vi "ClassPanel.vi"(8 "error in (no error)":errorcluster caption="entrée d'erreur (pas d'erreur)", 11 "AndorSpectro.lvclass":refnum<class "AndorSpectro.lvclass">) -> (0 "error out":errorcluster caption="sortie d'erreur", 3 "AndorSpectro.lvclass Out":refnum<class "AndorSpectro.lvclass">)   [LabVIEW 2019, in "AndorSpectro.lvclass"]
uses:
  AndorSpectro.lvclass
  C:/Programmes Labview/LabscanV1A/DevicesClass/BaseDevice/BaseDevice.lvclass
  <userlib>/ATSpectrograph/GUI/AndorNoiseCorr.ctl
  <userlib>/atmcd32d.llb/AndorCapabilities typedef.ctl
  <userlib>/atmcd32d.llb/Shutter_type typedef.ctl
  <userlib>/atmcd32d.llb/Shutter_mode typedef.ctl
  <userlib>/atmcd32d.llb/AcquisitionMode_mode typedef.ctl
  <userlib>/atmcd32d.llb/ReadMode_mode typedef.ctl
  <userlib>/atmcd32d.llb/Error Code Enum typedef.ctl
  BaseDevice/BaseDevice.lvclass/BaseDevice.ctl
  <userlib>/atmcd32d.llb/TriggerMode_mode typedef.ctl
  BaseDevice/ClassQueueMess.ctl
  <userlib>/atmcd32d.llb/HSSpeed_type typedef.ctl
  AndorSpectro.lvclass/AndorSpectro.ctl
  BaseDevice/Accessor/GetBaseDataPath.vi
  BaseDevice/Accessor/GetClassEvent.vi
  <userlib>/ATSpectrograph/atspectrograph.lvlib
panel:
  out "exposure":sgl format="%.4f"
  out "Top Wl":sgl=100.0 caption="Top Wl. (nm)" min=0 max=3000 step=0.01
  out "Bot Wl":sgl=100.0 caption="Bot Wl. (nm)" min=0 max=3000 step=0.01
  out "BaseDataPath":path
  out "Background":i32[][](array[numeric])
  out "AndorMainQ":refnum<queue>
  out "Wavelength":sgl
  out "CalValues":sgl[](array[numeric])
  out "Detector offset":i32
  out "grating out":i32
  out "Grating offset":i32
  out "gain":sgl format="%.2f"
  out "information":i32
  out "caps":T1
  in  "X Start":i32=1 min=1 max=1023 step=1
  in  "X End":i32=1024 min=2 max=1024 step=1
  in  "AndorTabs":enum32{"Main Controls", "Settings", "Data"}(tab)
  in  "Shutter":bool
  in  "DIsOnCLose":bool=TRUE caption="Dis.On Close"
  in  "AccDone":u16 caption="Acq. Done"
  in  "Stop Acq":bool
  in  "Con/Disc.":bool
  in  "Gain":i32(ring) caption="Device Name" items=["1.0(x)", "1.7(x)"]
  in  "Image Mode":bool
  in  "AquireImage":bool caption="MiseAJour"
  out "AcqTime":sgl caption="Acq. Time (s)" format="%#.4f"
  in  "IntegTime":u32=100 caption="Integration\nTime (ms)" min=1 max=100000 step=1
  in  "Accumulation":u16=1 min=1 max=256 step=1
  out "Temp °C":i32
  in  "Cooler":bool
  in  "Save Data":bool caption="Save\nData"
  in  "Cont. Acq.":bool caption="Cont.Acq."
  out "Stable":bool
  in  "Setp. °C":i32=-80
  out "Aquiring":bool
  in  "Save Bckgnd":bool caption="Save as \nBckgnd"
  in  "Backgnd Mode":T2
  in  "SetAreas":bool caption="MiseAJour"
  in  "Y Bins":i32=1 min=1 max=256 step=1
  out "areas":i32[][](array[numeric])=[[1], [1], [1], [1024], [256], [1], [256]]
  in  "HS":u16(ring) caption="Hor. Spd." items=["100kHz@16bit", "50kHz@16bit", "33kHz@16bit"]
  in  "VS":u16(ring)=1 caption="Vert. Spd (us)" items=["[8.25]", "16.25", "32.25", "64.25"]
  in  "Y End":i32=256 min=2 max=256 step=1
  in  "Y Start":i32=1 min=1 max=255 step=1
  in  "ShutterMode":u16(ring) items=["IDUS_Shutter", "Ext Shutter"]
  out "Start(nm)":sgl=1.0 min=1 max=255 step=1
  out "End(nm)":sgl=1.0 min=1 max=255 step=1
  out "WaveBands":T3(array[cluster]) {"WB End" min=1 max=255 step=1; "WB Start" min=1 max=255 step=1}
  in  "DelWB":bool caption="MiseAJour"
  in  "AddWB":bool caption="MiseAJour"
  in  "WB End":i32=256 min=2 max=1024 step=1
  in  "WB Start":i32=1 min=1 max=1023 step=1
  in  "NoiseWindow":bool caption="Noise Window"
  in  "Cosmic Filter":bool
  in  "MainProgQ":refnum<queue>
  in  "MainProgQEvent":refnum<user-event>
  in  "Acq":bool
  in  "Stop":bool
  out "Init Program":bool
  # "Andor Camera"
  # "this MUST labeled with class name"
  # "this MUST be present and labeled \"Stop\" and \"Acq\""
  # "Single Acq"
  # "Area#"
  # "X Origin"
  # "Y Origin"
  # "X Size"
  # "Y Size"
  # "X Bin"
  # "Y Bin"
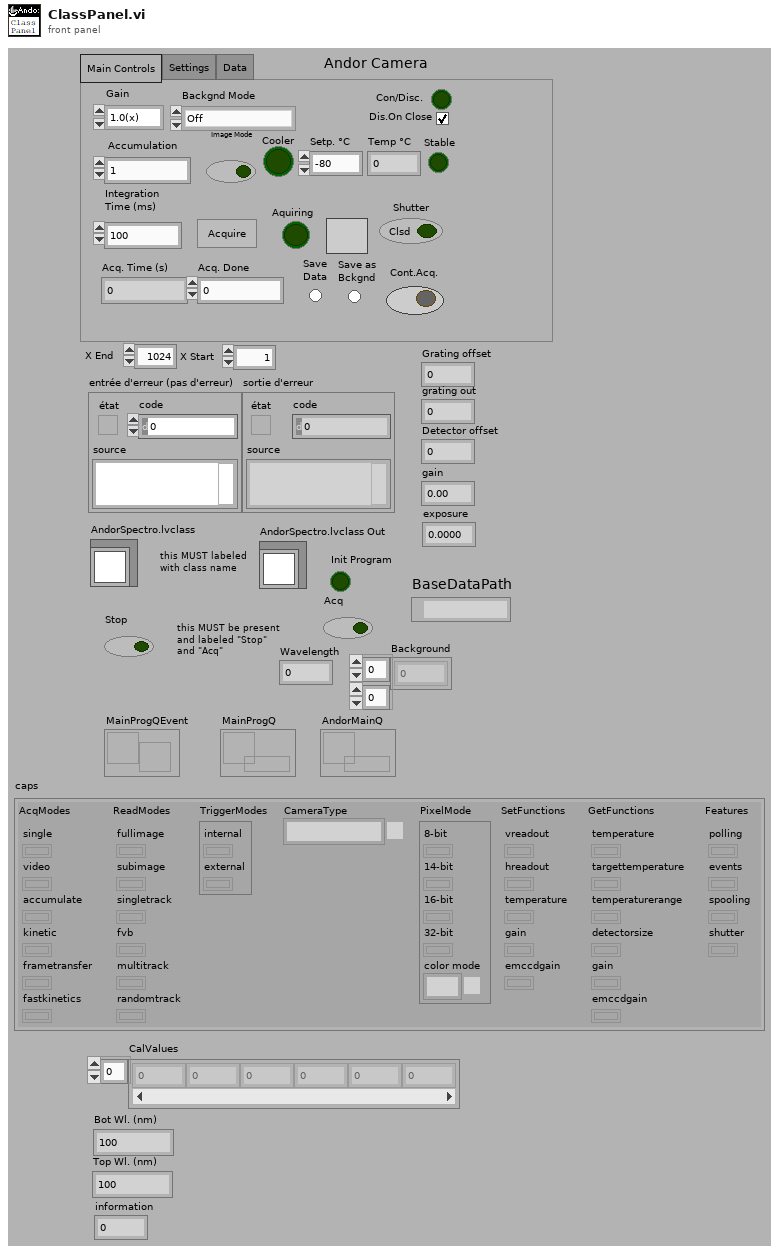
[diagram p1: front panel]
types:
  T1 = typedef "AndorCapabilities typedef.ctl" = cluster{"AcqModes":cluster{"single":bool, "video":bool, "accumulate":bool, "kinetic":bool, "frametransfer":bool, "fastkinetics":bool}, "ReadModes":cluster{"fullimage":bool, "subimage":bool, "singletrack":bool, "fvb":bool, "multitrack":bool, "randomtrack":bool}, "TriggerModes":cluster{"internal":bool, "external":bool}, "CameraType":enum32{"PDA", "iXon", "ICCD", "EMCCD", "CCD", "iStar", "third party camera", "iDus", "Newton", "Surcam", "USB ICCD", "Luca", "Reserved", "iKon", "InGaAs", "iVac", "Unprogrammed", "Clara", "USB iStar", "SimCam", "Neo", "iXon Ultra", "Volmos", "iVac Ultra"}, "PixelMode":cluster{"8-bit":bool, "14-bit":bool, "16-bit":bool, "32-bit":bool, "color mode":enum16{"Mono", "RGB", "CMY"}}, "SetFunctions":cluster{"vreadout":bool, "hreadout":bool, "temperature":bool, "gain":bool, "emccdgain":bool}, "GetFunctions":cluster{"temperature":bool, "targettemperature":bool, "temperaturerange":bool, "detectorsize":bool, "gain":bool, "emccdgain":bool}, "Features":cluster{"polling":bool, "events":bool, "spooling":bool, "shutter":bool}}
  T2 = typedef "AndorNoiseCorr.ctl" = enum16{"Off", "Selected Curve", "One For Every Acq"}
  T3 = cluster{"WB Start":i32, "WB End":i32, "Active":bool}[]
  T4 = cluster{"Message":string, "Data":variant, "Code":i32}
  T5 = typedef "Shutter_mode typedef.ctl" = enum16{"Auto", "Open", "Close", "N/A (3)", "Open FVB Series", "Open Any Series"}
  T6 = typedef "Shutter_type typedef.ctl" = enum16{"TTL Low", "TTL High"}
  T7 = typedef "AcquisitionMode_mode typedef.ctl" = enum16{"Reserved (0)", "Single Scan", "Accumulate", "Kinetics", "Fast Kinetics", "Run Till Abort", "Reserved (6)", "Reserved (7)", "Reserved (8)", "Time Delayed Integration"}
  T8 = typedef "ReadMode_mode typedef.ctl" = enum16{"Full Vertical Binning", "Multi-Track", "Random-Track", "Single-Track", "Image"}
  T9 = typedef "Error Code Enum typedef.ctl" = enum32{"N/A (0)", "DRV_ERROR_CODES", "DRV_SUCCESS", "DRV_VXDNOTINSTALLED", "DRV_ERROR_SCAN", "DRV_ERROR_CHECK_SUM", "DRV_ERROR_FILELOAD", "DRV_UNKNOWN_FUNC", "DRV_ERROR_VXD_INIT", "DRV_ERROR_ADDRESS", "DRV_ERROR_PAGELOCK", "DRV_ERROR_PAGEUNLOCK", "DRV_ERROR_BOARDTEST", "DRV_ERROR_ACK", "DRV_ERROR_UP_FIFO", "DRV_ERROR_PATTERN", "N/A (16)", "DRV_ACQUISITION_ERRORS", "DRV_ACQ_BUFFER", "DRV_ACQ_DOWNFIFO_FULL", "DRV_PROC_UNKONWN_INSTRUCTION", "DRV_ILLEGAL_OP_CODE", "DRV_KINETIC_TIME_NOT_MET", "DRV_ACCUM_TIME_NOT_MET", "DRV_NO_NEW_DATA", "N/A (25)", "DRV_SPOOLERROR", "N/A (27)", "N/A (28)", "N/A (29)", "N/A (30)", "N/A (31)", "N/A (32)", "DRV_TEMPERATURE_CODES", "DRV_TEMPERATURE_OFF", "DRV_TEMPERATURE_NOT_STABILIZED", "DRV_TEMPERATURE_STABILIZED", "DRV_TEMPERATURE_NOT_REACHED", "DRV_TEMPERATURE_OUT_RANGE", "DRV_TEMPERATURE_NOT_SUPPORTED", "DRV_TEMPERATURE_DRIFT", "N/A (41)", "N/A (42)", "N/A (43)", "N/A (44)", "N/A (45)", "N/A (46)", "N/A (47)", "N/A (48)", "DRV_GENERAL_ERRORS", "DRV_INVALID_AUX", "DRV_COF_NOTLOADED", "DRV_FPGAPROG", "DRV_FLEXERROR", "DRV_GPIBERROR", "N/A (55)", "N/A (56)", "N/A (57)", "N/A (58)", "N/A (59)", "N/A (60)", "N/A (61)", "N/A (62)", "N/A (63)", "DRV_DATATYPE", "DRV_DRIVER_ERRORS", "DRV_P1INVALID", "DRV_P2INVALID", "DRV_P3INVALID", "DRV_P4INVALID", "DRV_INIERROR", "DRV_COFERROR", "DRV_ACQUIRING", "DRV_IDLE", "DRV_TEMPCYCLE", "DRV_NOT_INITIALIZED", "DRV_P5INVALID", "DRV_P6INVALID", "DRV_INVALID_MODE", "DRV_INVALID_FILTER", "DRV_I2CERRORS", "DRV_I2CDEVNOTFOUND", "DRV_I2CTIMEOUT", "DRV_P7INVALID", "N/A (84)", "N/A (85)", "N/A (86)", "N/A (87)", "N/A (88)", "N/A (89)", "DRV_IOCERROR", "DRV_VRMVERSIONERROR"}
  T10 = typedef "HSSpeed_type typedef.ctl" = enum16{"EM Amp", "Conventional Amp"}
  T11 = typedef "TriggerMode_mode typedef.ctl" = enum16{"Internal", "External", "N/A (2)", "N/A (3)", "N/A (4)", "N/A (5)", "External Start"}
  T12 = typedef "ClassQueueMess.ctl" = u16
  T13 = cluster{"wavelength out":sgl, "calibrationValuesOut":sgl[], "gain":sgl, bool}
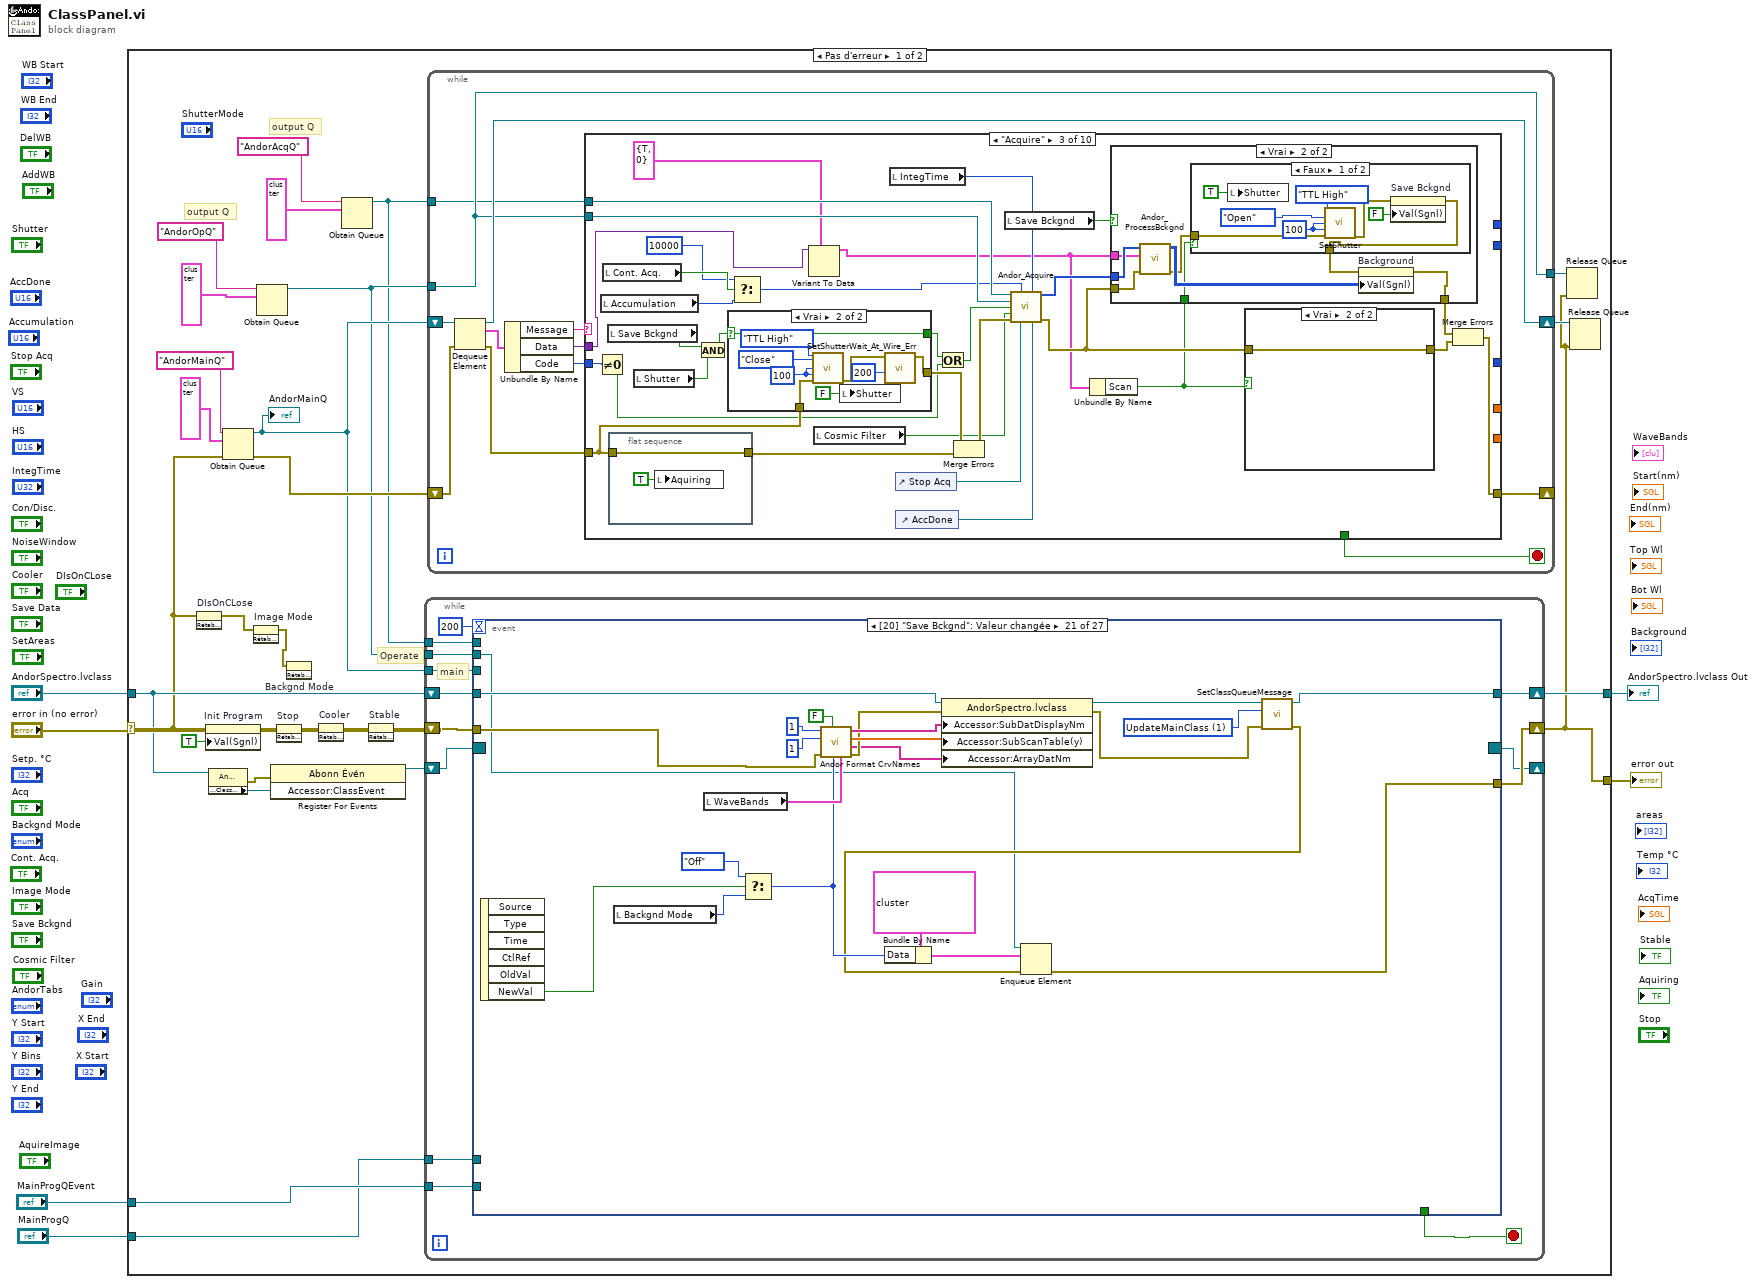
[diagram p0: block diagram]
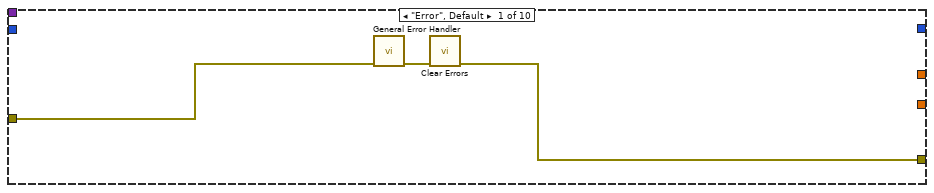
[diagram p2: hidden frame]
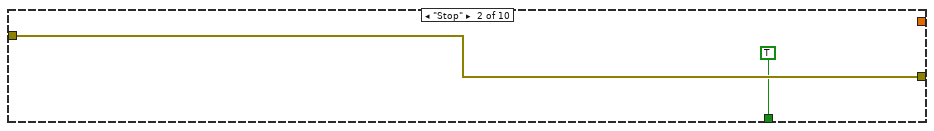
[diagram p3: hidden frame]
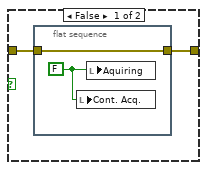
[diagram p4: hidden frame]
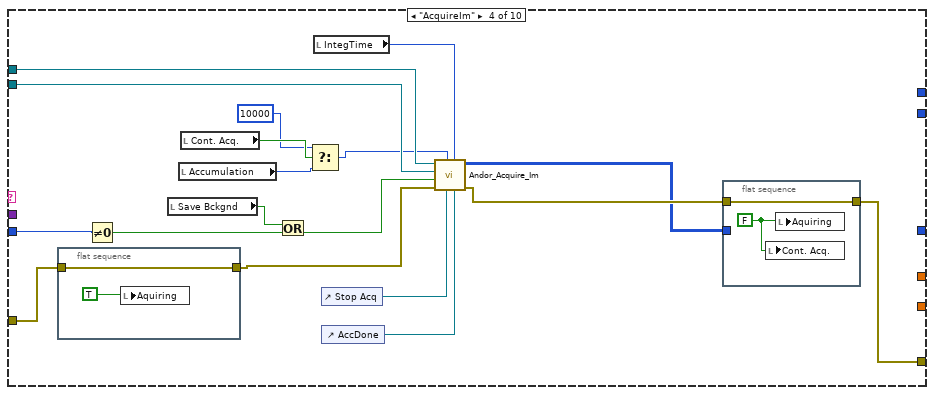
[diagram p8: hidden frame]
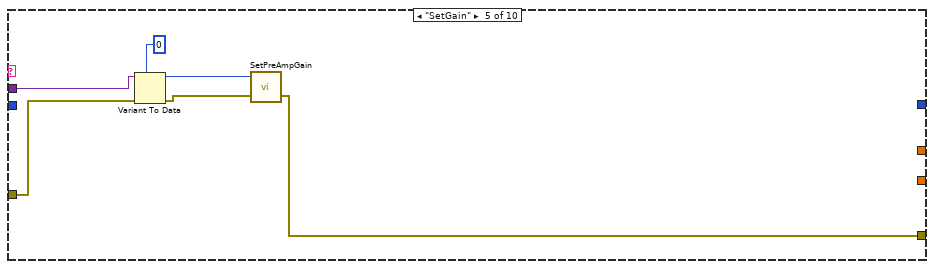
[diagram p9: hidden frame]
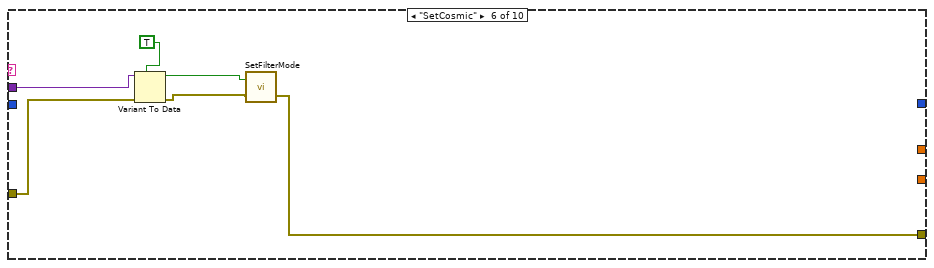
[diagram p10: hidden frame]
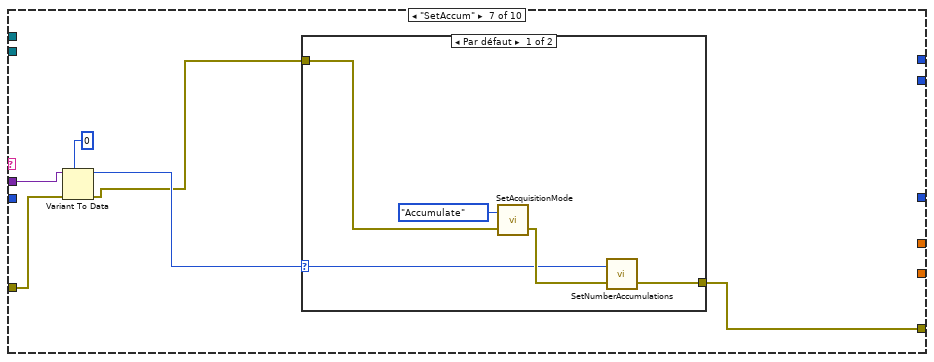
[diagram p11: hidden frame]
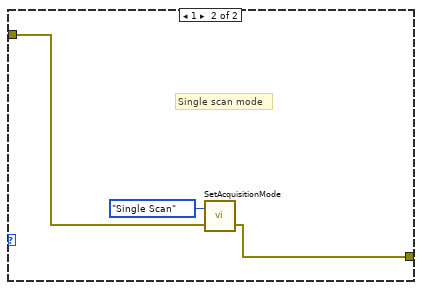
[diagram p12: hidden frame]
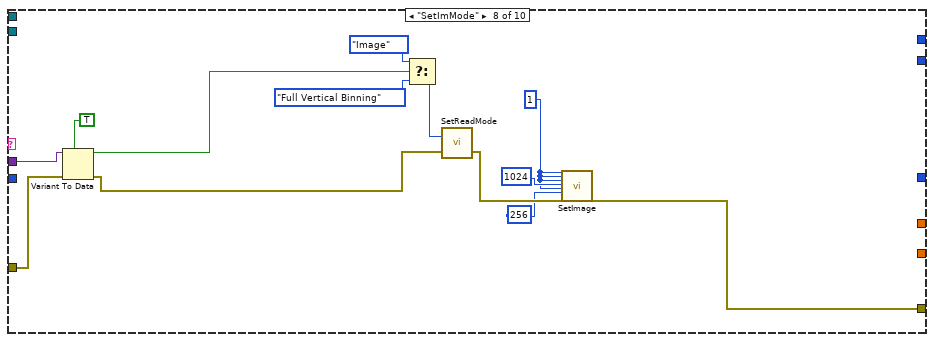
[diagram p13: hidden frame]
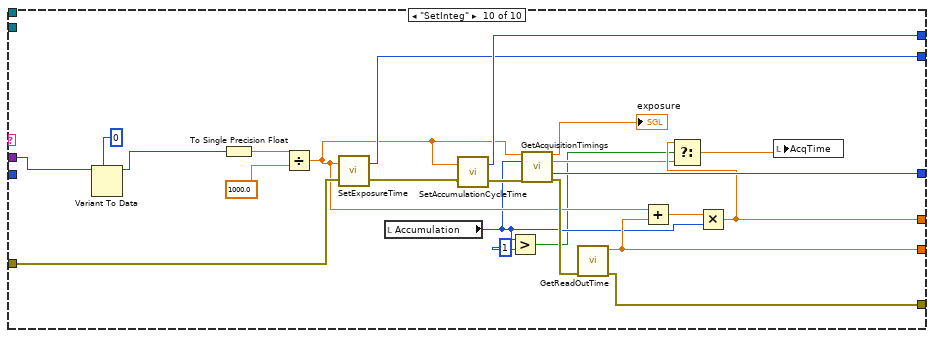
[diagram p15: hidden frame]
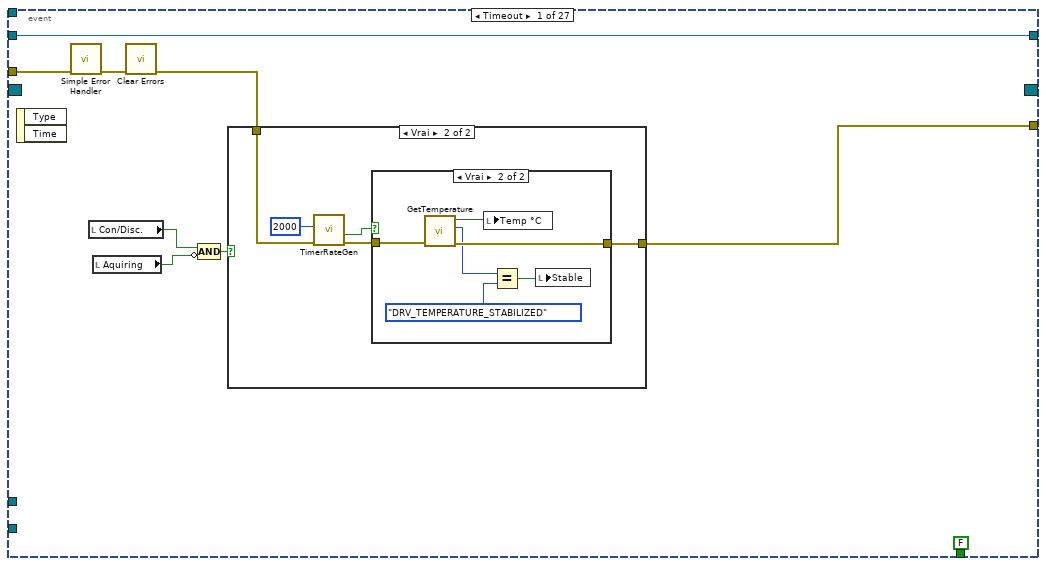
[diagram p16: hidden frame]
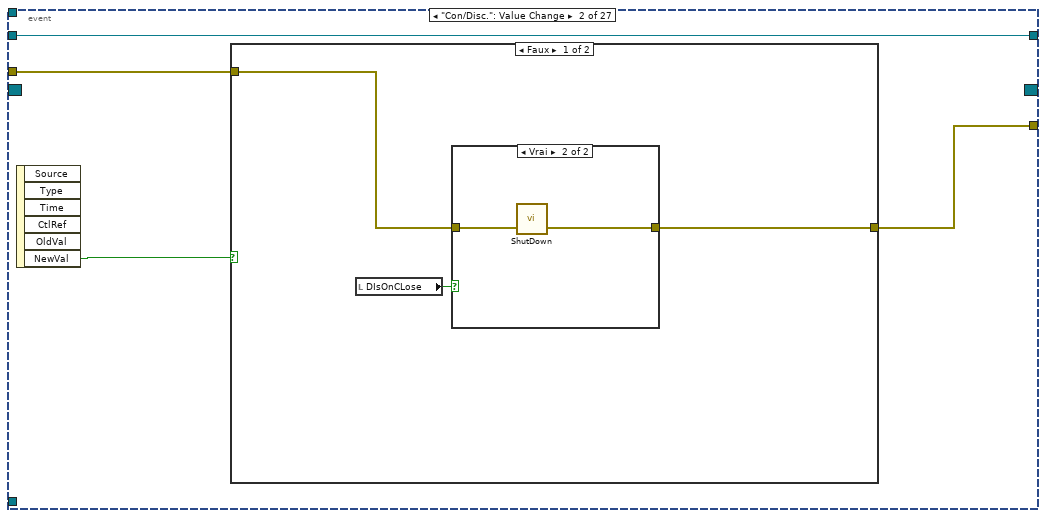
[diagram p19: hidden frame]
diagram:
  n1 = case shown="Pas d'erreur" "error in (no error)" {
    selector: "error in (no error)" -> [w11 w800]
    tunnel: [w8 w800] -> w5
    tunnel: "AndorSpectro.lvclass" -> [w29 w799]
    tunnel: [w33 w799] -> w3
    tunnel: "MainProgQEvent" -> [w27 _]
    tunnel: "MainProgQ" -> [w26 _]
    frame No Error {
      # "Operate"
      # "output Q"
      # "output Q"
      n2 = invoke on="DIsOnCLose" class="Bool (strict)" method="RétablirValParDéfaut"(error in=w11) -> (error out=w10:errorcluster)  [unwired: 2 in, 2 out]
      n3 = property on="Init Program" class="Bool (strict)"(error in=w11, "Val(Sgnl)"=TRUE ("Valeur (Signalisation)")) -> (error out=w32:errorcluster)  [unwired: 1 in, 1 out]
      n4 = property class="AndorSpectro.lvclass"(reference=w29) -> (error out=w31:errorcluster, "Accessor:ClassEvent"=w30:refnum<user-event>)  [unwired: 1 in, 1 out]
      n5 = Obtain Queue(name (unnamed)="AndorMainQ" ("nom (aucun)"), element data type=T4 {"Message"="", "Data"=variant, "Code"=0}, error in (no error)=w11) -> (queue out=w22:refnum<queue>, error out=w24:errorcluster)  [unwired: 2 in, 1 out]
      "AndorMainQ" <- w22
      n6 = invoke on="Image Mode" class="Bool (strict)" method="RétablirValParDéfaut"(error in=w10) -> (error out=w7:errorcluster)  [unwired: 2 in, 2 out]
      n7 = Obtain Queue(name (unnamed)="AndorOpQ" ("nom (aucun)"), element data type=T4 {"Message"="", "Data"=variant, "Code"=0} ("element")) -> (queue out=w17:refnum<queue>)  [unwired: 3 in, 2 out]
      n8 = register-events(error in=w31, w30) -> (reference out=w28:refnum<event-registration>)  [unwired: 1 in, 1 out]
      n9 = invoke on="Stop" class="Bool (strict)" method="RétablirValParDéfaut"(error in=w32) -> (error out=w18:errorcluster)  [unwired: 2 in, 2 out]
      n10 = invoke on="Backgnd Mode" class="Énum (strict)" method="RétablirValParDéfaut"(error in=w7) -> ()  [unwired: 2 in, 3 out]
      n11 = invoke on="Cooler" class="Bool (strict)" method="RétablirValParDéfaut"(error in=w18) -> (error out=w13:errorcluster)  [unwired: 2 in, 2 out]
      n12 = Obtain Queue(name (unnamed)="AndorAcqQ" ("nom (aucun)"), element data type=T4 {"Message"="", "Data"=variant, "Code"=0} ("element")) -> (queue out=w14:refnum<queue>)  [unwired: 3 in, 2 out]
      n13 = invoke on="Stable" class="Bool (strict)" method="RétablirValParDéfaut"(error in=w13) -> (error out=w12:errorcluster)  [unwired: 2 in, 2 out]
      n14 = while {
        shift-right: [w214] -> w8
        shift-left: w12 -> [w215]
        shift-right: [w212] -> w33
        shift-left: w29 -> [w213]
        shift-right: [w210] -> _
        shift-left: w28 -> [w211]
        tunnel: w27 -> [w209]
        tunnel: w26 -> [w208]
        tunnel: w22 -> [w207]
        tunnel: w17 -> [w206]
        tunnel: w14 -> [w205]
        stop <- w204 stop-if-true
        # "main"
        n15 = event shown="[20] \"Save Bckgnd\": Valeur changée" {
          selector: w211 -> [_ _ _ _ _ _ _ _ _ _ _ _ _ _ _ _ _ _ _ _ _ _ _ _ _ _ _]
          dyn-events: [_ _ _ _ _ _ _ _ _ _ _ _ _ _ _ _ _ _ _ _ _ _ _ _ _ _ _] -> w210
          timeout: 200 -> [_ _ _ _ _ _ _ _ _ _ _ _ _ _ _ _ _ _ _ _ _ _ _ _ _ _ _]
          tunnel: w215 -> [w223 w241 w264 w295 w331 w335 w347 w366 w381 w390 w498 w505 w523 w527 w558 w574 w598 w602 w641 w647 w665 w693 w695 w708 w717 w765 w795]
          tunnel: [w219 w239 w258 w293 w330 w335 w346 w365 w381 w384 w493 w503 w521 w532 w557 w573 w595 w603 w642 w646 w655 w678 w694 w702 w713 w764 w790] -> w214
          tunnel: w213 -> [w224 w240 w265 w297 w332 w336 w344 w363 w382 w387 w500 w506 w520 w535 w571 w575 w599 w605 w639 w654 w667 w692 w697 w710 w718 w766 w798]
          tunnel: [FALSE _ _ TRUE _ _ _ _ _ FALSE _ _ _ _ _ _ _ _ _ _ _ _ _ _ _ _ _] -> w204
          tunnel: [w224 w240 w257 w297 w332 w336 w345 w364 w382 w386 w500 w506 w520 w535 w556 w575 w599 w605 w638 w654 w666 w691 w697 w710 w714 w766 w798] -> w212
          tunnel: w209 -> [_ _ w256 _ _ _ _ _ _ _ _ _ _ _ _ _ _ _ _ _ _ _ _ _ w715 _ _]
          tunnel: w208 -> [_ _ w255 _ _ _ _ _ _ _ _ _ _ _ _ _ _ _ _ _ _ _ _ _ w716 _ _]
          tunnel: w207 -> [_ _ _ w296 _ _ _ _ _ w388 _ _ _ w524 w565 w572 _ _ _ _ _ _ _ w709 w712 _ w794]
          tunnel: w206 -> [_ _ _ w294 w329 _ _ _ _ w389 w492 _ _ _ _ _ w597 _ w643 _ w656 _ _ w704 w711 _ w793]
          tunnel: w205 -> [_ _ _ _ _ _ _ _ _ w385 _ _ _ _ _ _ _ _ _ _ _ _ _ _ _ _ _]
          event Timeout {
            n16 = event-data() -> ()  [unwired: 1 in, 2 out]
            n17 = call <vilib>:"Simple Error Handler.vi"("error in (no error)"=w223) -> ("error out"=w222:errorcluster)  [unwired: 4 in, 4 out]
            n18 = local read "Con/Disc."() -> (w221:bool)
            n19 = local read "Aquiring"() -> (w217:bool)
            n20 = call <vilib>:"Clear Errors.vi"("error in (no error)"=w222) -> ("error out"=w220:errorcluster)  [unwired: 5 in, 1 out]
            n21 = Compound Arithmetic op=AND ("Opérateur arithmétique")(w221, invert w217) -> (w218:bool)
            n22 = case shown="Vrai" w218 {
              tunnel: w220 -> [w226 w230]
              tunnel: [w226 w228] -> w219
              frame False {
              }
              frame True {
                n23 = call <userlib>:"TimerRateGen.vi"("error in (no error)"=w230, "Refresh(ms)"=u32 2000) -> ("error out"=w229:errorcluster, "updated?"=w227:bool)  [unwired: 7 in, 1 out]
                n24 = case shown="Vrai" w227 {
                  tunnel: w229 -> [w232 w238]
                  tunnel: [w232 w236] -> w228
                  frame False {
                  }
                  frame True {
                    n25 = call <userlib>:"GetTemperature.vi"("error in (no error)"=w238) -> ("error out"=w236:errorcluster, "status"=w235:T9, "temperature"=w237:i32)  [unwired: 3 in, 1 out]
                    n26 = local write "Temp °C"(w237) -> ()
                    n27 = Equal?(x=w235, y=Error_Code_Enum_typedef."DRV_TEMPERATURE_STABILIZED" ("status")) -> (x = y?=w233:bool)
                    n28 = local write "Stable"(w233) -> ()
                  }
                }
              }
            }
          }
          event "Con/Disc.": Value Change {
            n29 = event-data() -> ("NewVal"=w242:bool)  [unwired: 1 in, 5 out]
            n30 = case shown="Faux" w242 {
              tunnel: w241 -> [w245 w253]
              tunnel: [w244 w252] -> w239
              frame False {
                n31 = local read "DIsOnCLose"() -> (w243:bool)
                n32 = case shown="Vrai" w243 {
                  tunnel: w245 -> [w246 w248]
                  tunnel: [w246 w247] -> w244
                  frame False {
                  }
                  frame True {
                    n33 = call <userlib>:"ShutDown.vi"("error in (no error)"=w248) -> ("error out"=w247:errorcluster)  [unwired: 1 in, 1 out]
                  }
                }
              }
              frame True {
                n34 = property on="Init Program" class="Bool (strict)"(error in=w253, "Val(Sgnl)"=TRUE ("Valeur (Signalisation)")) -> (error out=w252:errorcluster)  [unwired: 1 in, 1 out]
                n35 = call <userlib>:"Wait_At_Wire_Bool.vi"("Wait (ms)"=u32 300, "error in (no error)"=FALSE ("Con/Disc.")) -> ("error out"=w250:bool)  [unwired: 7 in, 2 out]
                n36 = local write "Con/Disc."(w250) -> ()
              }
            }
          }
          event User Event {
            n37 = event-data() -> ("queue out"=w262:refnum<queue>)  [unwired: 1 in, 3 out]
            n38 = Dequeue Element(queue=w262) -> (element=w263:cluster{"Message":string, "Data":variant, i32})  [unwired: 2 in, 3 out]
            n39 = Unbundle(w263) -> ("Message"=w261:string, "Data"=w260:variant, w259:i32)
            n40 = case shown="\"UpdateMainClass\"" w261 {
              tunnel: w264 -> [w267 w272 w276 w277 w281 w284]
              tunnel: w260 -> [_ w271 w275 _ _ _]
              tunnel: w265 -> [w266 w270 w274 w278 w282 w287]
              tunnel: [w266 w269 w273 w278 w282 w287] -> w257
              tunnel: [w267 w272 w276 w277 w281 w283] -> w258
              tunnel: w259 -> [_ _ _ _ _ _]
              tunnel: w256 -> [_ _ _ _ _ w286]
              tunnel: w255 -> [_ _ _ _ _ w285]
              frame Default {
              }
              frame "UpdateClassData" {
                n41 = Variant To Data(type=w270, Variant=w271) -> (data=w269:refnum<class "AndorSpectro.lvclass">)  [unwired: 1 in, 1 out]
                n42 = property class="AndorSpectro.lvclass"(reference=w269) -> ("Accessor:BaseDataPath"=→"BaseDataPath":path)  [unwired: 1 in, 2 out]
              }
              frame "UpdateDataBind" {
                n43 = Variant To Data(type=w274, Variant=w275) -> (data=w273:refnum<class "AndorSpectro.lvclass">)  [unwired: 1 in, 1 out]
              }
              frame "MeasDone" {
              }
              frame "ShowDiag" {
                n44 = control-ref of="This VI"() -> (w280:refnum<vi>)
                n45 = call <userlib>:"AnimExecGen.vi"("Animer l'exécution ?"=TRUE, "ViRef"=w280) -> ()  [unwired: 9 in, 1 out]
              }
              frame "UpdateMainClass" {
                n46 = Bundle By Name(cluster=cluster{"Message":string, "Data":variant, i32} {"Message"="", "Data"=variant, 0} ("élément"), "Data"=w287) -> (w288:cluster{"Message":string, "Data":variant, i32})
                n47 = Enqueue Element(queue=w285, element=w288, error in (no error)=w284) -> (queue out=w291:refnum<queue>, error out=w290:errorcluster)  [unwired: 1 in, 1 out]
                n48 = Generate User Event(user event=w286, event data cluster=w291, error in=w290) -> (error out=w283:errorcluster)  [unwired: 1 in, 1 out]
              }
            }
          }
          event "Stop": Value Change {
            n49 = event-data() -> ("NewVal"=w292:bool)  [unwired: 1 in, 5 out]
            n50 = case shown="Vrai" w292 {
              tunnel: w296 -> [_ w302]
              tunnel: w295 -> [w299 w309]
              tunnel: w294 -> [_ w306]
              tunnel: [w299 w305] -> w293
              frame False {
              }
              frame True {
                w300 = T4 {"Message"="Stop", "Data"=variant, "Code"=0} ("élément")
                n51 = local read "DIsOnCLose"() -> (w303:bool)
                n52 = Enqueue Element(queue=w302, element=w300, error in (no error)=w309) -> (error out=w301:errorcluster)  [unwired: 1 in, 2 out]
                n53 = case shown="Faux" w303 {
                  tunnel: [w311 w318] -> w308
                  tunnel: w306 -> [w313 w317]
                  tunnel: w301 -> [w312 w315]
                  tunnel: w300 -> [_ w314]
                  frame False {
                    n54 = Enqueue Element(queue=w313, element=T4 {"Message"="Standalone", "Data"=variant, "Code"=0} ("élément"), error in (no error)=w312) -> (error out=w311:errorcluster)  [unwired: 1 in, 2 out]
                  }
                  frame True {
                    n55 = Enqueue Element(queue=w317, element=w314, error in (no error)=w315) -> (error out=w316:errorcluster)  [unwired: 1 in, 2 out]
                    n56 = call <userlib>:"ShutDown.vi"("error in (no error)"=w316) -> ("error out"=w318:errorcluster)  [unwired: 1 in, 1 out]
                  }
                }
                n57 = call <userlib>:"AT Spectrograph Close.vi"("error in (no error)"=w308) -> ("error out"=w307:errorcluster)  [unwired: 9 in, 1 out]
                n58 = call <userlib>:"Wait_At_Wire_Err.vi"("Wait (ms)"=u32 300, "error in (no error)"=w307) -> ("error out"=w305:errorcluster)  [unwired: 7 in, 2 out]
              }
            }
          }
          event "CalValues": Value Change {
            n59 = event-data() -> ("NewVal"=w327:sgl[])  [unwired: 1 in, 5 out]
            n60 = local read "WB Start"() -> (w324:i32)
            n61 = local read "WB End"() -> (w323:i32)
            n62 = Decrement(x=w323) -> (x-1=w321:i32)
            n63 = Decrement(x=w324) -> (x-1=w322:i32)
            n64 = Index Array(array=w327, index #1=0 ("indice"), index #2=w322, index #3=w321) -> (element #1=w328:sgl, element #2=w320:sgl, element #3=w319:sgl)
            n65 = Delete From Array(array=w327) -> (deleted portion=w326:sgl)  [unwired: 2 in, 1 out]
            n66 = local write "Top Wl"(w326) -> ()
            n67 = local write "End(nm)"(w319) -> ()
            n68 = local write "Start(nm)"(w320) -> ()
            n69 = local write "Bot Wl"(w328) -> ()
            n70 = Bundle By Name(cluster=T4 {"Message"="UpdateWl", "Data"=variant, "Code"=1}, "Data"=w327) -> (w334:T4)
            n71 = Enqueue Element(queue=w329, element=w334, error in (no error)=w331) -> (error out=w330:errorcluster)  [unwired: 1 in, 2 out]
          }
          event "WB End", "WB Start": Value Change {
            n72 = event-data() -> ()  [unwired: 1 in, 6 out]
            n73 = local read "CalValues"() -> (w340:sgl[])
            n74 = local read "WB Start"() -> (w343:i32)
            n75 = local read "WB End"() -> (w342:i32)
            n76 = Decrement(x=w342) -> (x-1=w339:i32)
            n77 = Decrement(x=w343) -> (x-1=w341:i32)
            n78 = Index Array(array=w340, index #1=w341, index #2=w339) -> (element #1=w338:sgl, element #2=w337:sgl)
            n79 = local write "End(nm)"(w337) -> ()
            n80 = local write "Start(nm)"(w338) -> ()
          }
          event "AddWB": Value Change {
            n81 = event-data() -> ("NewVal"=w348:bool)  [unwired: 1 in, 5 out]
            n82 = case shown="Vrai" w348 {
              tunnel: [w350 w351] -> w346
              tunnel: w347 -> [w350 w352]
              tunnel: [w349 w354] -> w345
              tunnel: w344 -> [w349 w354]
              frame False {
              }
              frame True {
                n83 = local read "WaveBands"() -> (w359:T3)
                n84 = local read "WB End"() -> (w361:i32)
                n85 = local read "WB Start"() -> (w362:i32)
                n86 = Bundle("WB Start"=w362, "WB End"=w361, TRUE) -> (w358:cluster{"WB Start":i32, "WB End":i32, bool})  [unwired: 1 in]
                n87 = Insert Into Array(array=w359, new element=w358) -> (w353:T3)  [unwired: 1 in]
                n88 = property on="WaveBands" class="Tabl (strict)"(error in=w352, "Val(Sgnl)"=w353) -> (error out=w351:errorcluster)  [unwired: 1 in, 1 out]
                n89 = call <userlib>:"Wait_At_Wire_Bool.vi"("Wait (ms)"=u32 300, "error in (no error)"=FALSE) -> ("error out"=w357:bool)  [unwired: 7 in, 2 out]
                n90 = local write "AddWB"(w357) -> ()
              }
            }
          }
          event "DelWB": Value Change {
            n91 = event-data() -> ("NewVal"=w367:bool)  [unwired: 1 in, 5 out]
            n92 = case shown="Vrai" w367 {
              tunnel: [w369 w373] -> w365
              tunnel: w366 -> [w369 w374]
              tunnel: [w368 w376] -> w364
              tunnel: w363 -> [w368 w376]
              frame False {
              }
              frame True {
                n93 = local read "WaveBands"() -> (w380:T3)
                n94 = property on="WaveBands" class="Tabl (strict)"() -> ("Index Values"=w372:u32[])  [unwired: 2 in, 2 out]
                n95 = Index Array(array=w372) -> (element=w370:u32)  [unwired: 1 in]
                n96 = Delete From Array(array=w380, length=1 ("longueur"), index=w370) -> (array with subset deleted=w375:T3)  [unwired: 1 out]
                n97 = property on="WaveBands" class="Tabl (strict)"(error in=w374, "Val(Sgnl)"=w375) -> (error out=w373:errorcluster)  [unwired: 1 in, 1 out]
                n98 = call <userlib>:"Wait_At_Wire_Bool.vi"("Wait (ms)"=u32 300, "error in (no error)"=FALSE) -> ("error out"=w379:bool)  [unwired: 7 in, 2 out]
                n99 = local write "DelWB"(w379) -> ()
              }
            }
          }
          event Panel Close? {
            n100 = event-data() -> ()  [unwired: 1 in, 4 out]
            n101 = event-data("Discard?"=TRUE ("Rejeter ?")) -> ()  [unwired: 1 in, 1 out]
          }
          event "Init Program": Value Change {
            n102 = event-data() -> ("NewVal"=w392:bool)  [unwired: 1 in, 4 out]
            n103 = case shown="Vrai" w392 {
              tunnel: w390 -> [w394 w408]
              tunnel: [w394 w409] -> w384
              tunnel: [_ w455] -> _
              tunnel: [_ w454] -> _
              tunnel: [_ w451] -> _
              tunnel: [_ w437] -> _
              tunnel: w389 -> [_ w431]
              tunnel: w388 -> [_ w426]
              tunnel: w387 -> [w393 w432]
              tunnel: [w393 w428] -> w386
              tunnel: w385 -> [_ w427]
              frame False {
              }
              frame True {
                w399 = 100 ("closingtime")
                w418 = 0 ("index")
                w412 = u16 1 items=["[8.25]", "16.25", "32.25", "64.25"] ("VS")
                w420 = 1 items=["Gain  1.0(x)", "Gain  1.7(x)"] ("Gain")
                w429 = T12 1 items=["UpdateClassData", "UpdateMainClass", "UpdateDataBind", "ReInitDevice", "Custom", "ClosePan"] ("Menu déroulant")
                w458 = u32 0 items=["DIRECT", "SIDE"] ("entrancePort")
                w459 = u32 0 items=["DIRECT", "SIDE"] ("exitPort")
                w445 = 0
                w447 = 0
                w483 = -80 ("temperature")
                w488 = u32 20002  # DRV_SUCCESS
                n104 = call <userlib>:"Initialize.vi"("error in (no error)"=w408, "directory (\"\")"="" ("directory (\"\")")) -> ("error out"=w477:errorcluster, "DLL error code"=w489:u32)
                n105 = local write "Image Mode"(FALSE ("Image Mode")) -> ()
                n106 = Initialize Array(0 ("élément"), 1024 ("numberPixels"), 1 ("taille de la dimension")) -> (w406:i32[][])
                n107 = call <userlib>:"Wait_At_Wire_Err.vi"("Wait (ms)"=u32 2000, "error in (no error)"=w477) -> ("error out"=w475:errorcluster)  [unwired: 7 in, 2 out]
                n108 = Equal?(x=w489, y=w488) -> (x = y?=w473:bool)
                n109 = Open VI Reference(type specifier VI Refnum (for type only)=refnum<vi> refnum ("référence"), vi path=path "C:/Program Files (x86)/National Instruments/LabVIEW 2019/user.lib/ATSpectrograph/GUI/Andor_Operate.vi" ("chemin du VI"), options=128, error in (no error)=w408) -> (vi reference=w422:refnum<vi>, error out=w421:errorcluster)  [unwired: 2 in]
                n110 = local write "Background"(w406) -> ()
                n111 = call <userlib>:"GetCameraInformation.vi"("error in (no error)"=w475) -> ("error out"=w476:errorcluster, "information"=w472:i32)  [unwired: 2 in, 1 out]
                "information" <- w472
                n112 = Equal?(x=7, y=w472) -> (x = y?=w470:bool)
                n113 = call-by-ref "Démarrer un appel asynchrone"(reference=w422, error in=w421, 8:"error in (no error)"=w408, "AndorAcqQ"=w426, "AndorOpQ"=w431) -> ()  [unwired: 8 in, 3 out]
                n114 = call <userlib>:"GetCapabilities.vi"("error in (no error)"=w476) -> ("error out"=w474:errorcluster, "caps"=→"caps":T1)  [unwired: 2 in, 1 out]
                n115 = And(x=w473, y=w470) -> (x .and. y?=w433:bool)
                n116 = local write "Con/Disc."(w433) -> ()
                n117 = local write "Setp. °C"(w483) -> ()
                n118 = property on="Accumulation" class="NumNb (strict)"("Value"=u16 1 ("Accumulation")) -> ()  [unwired: 2 in, 2 out]
                n119 = call <userlib>:"SetReadMode.vi"("error in (no error)"=w474, "mode"=ReadMode_mode_typedef."Full Vertical Binning") -> ("error out"=w485:errorcluster)  [unwired: 1 out]
                n120 = call <userlib>:"SetAcquisitionMode.vi"("error in (no error)"=w485, "mode"=AcquisitionMode_mode_typedef."Single Scan") -> ("error out"=w466:errorcluster)  [unwired: 1 out]
                n121 = Bundle By Name(cluster=w432, "AndorOpQ"=w431, "AndorAcqQ"=w427, "AndorMainQ"=w426) -> (w430:refnum<class "AndorSpectro.lvclass">)
                n122 = call <userlib>:"GetPreAmpGain.vi"("error in (no error)"=w466, "index"=0) -> ("gain"=w434:sgl)  [unwired: 1 in, 2 out]
                "gain" <- w434
                n123 = call <userlib>:"SetPreAmpGain.vi"("error in (no error)"=w466, "index"=w420) -> ("error out"=w411:errorcluster)  [unwired: 1 out]
                n124 = property on="Gain" class="MDér (strict)"(error in=w466, "Value"=w420) -> (error out=w480:errorcluster)  [unwired: 1 in, 1 out]
                n125 = property on="HS" class="MDér (strict)"(error in=w480, "Value"=w418) -> (error out=w479:errorcluster)  [unwired: 1 in, 1 out]
                n126 = property class="AndorSpectro.lvclass" props=["Accessor:DataBindCtrl", "Accessor:DataCtrl"](reference=w430) -> (reference out=w403:refnum<class "AndorSpectro.lvclass">)  [unwired: 1 in, 3 out]
                n127 = call <userlib>:"SetHSSpeed.vi"("error in (no error)"=w411, "index"=w418, "type"=HSSpeed_type_typedef."EM Amp") -> ("error out"=w410:errorcluster)  [unwired: 1 in, 1 out]
                n128 = local write "Shutter"(FALSE ("Shutter")) -> ()
                n129 = call <userlib>:"SetVSSpeed.vi"("error in (no error)"=w410, "index"=w412) -> ("error out"=w413:errorcluster)  [unwired: 1 out]
                n130 = property on="VS" class="MDér (strict)"(error in=w479, "Value"=w412) -> ()  [unwired: 1 in, 2 out]
                n131 = call <userlib>:"GetPixelSize.vi"("error in (no error)"=w413) -> ("error out"=w456:errorcluster, "ysize"=w454:sgl, "xsize"=w455:sgl)  [unwired: 3 in, 1 out]
                n132 = call <userlib>:"GetFilterMode.vi"("error in (no error)"=w456) -> ("error out"=w396:errorcluster, "mode"=w402:bool)  [unwired: 2 in, 1 out]
                n133 = call <userlib>:"SetShutter.vi"("type"=Shutter_type_typedef."TTL High", "mode"=Shutter_mode_typedef."Close", "closingtime"=w399, "openingtime"=w399, "error in (no error)"=w396) -> ("error out"=w398:errorcluster)  [unwired: 9 in, 1 out]
                n134 = call <userlib>:"SetTemperature.vi"("error in (no error)"=w398, "temperature"=w483) -> ("error out"=w417:errorcluster)  [unwired: 1 out]
                n135 = call <userlib>:"CoolerON.vi"("error in (no error)"=w417) -> ("error out"=w416:errorcluster)  [unwired: 1 in, 1 out]
                n136 = Unbundle By Name(w416) -> ("status"=w415:bool)
                n137 = Not(x=w415) -> (.not. x?=w414:bool)
                n138 = local write "Cooler"(w414) -> ()
                n139 = call <userlib>:"SetTriggerMode.vi"("error in (no error)"=w416, "mode"=TriggerMode_mode_typedef."Internal") -> ("error out"=w450:errorcluster)  [unwired: 1 out]
                n140 = property on="IntegTime" class="NumNb (strict)"(error in=w450, "Val(Sgnl)"=u32 100 ("Valeur (Signalisation)")) -> (error out=w453:errorcluster)  [unwired: 1 in, 1 out]
                n141 = call <userlib>:"AT Spectrograph Initialize.vi"("error in (no error)"=w453, "iniPath"="") -> ("error out"=w449:errorcluster, "function return"=w451:u32)  [unwired: 8 in]
                n142 = call <userlib>:"AT Spectrograph Get Wavelength.vi"("error in (no error)"=w449, "device"=w447) -> ("error out"=w448:errorcluster, "wavelength out"=w437:sgl)  [unwired: 7 in, 1 out]
                "Wavelength" <- w437
                n143 = call <userlib>:"AT Spectrograph Set Pixel Width.vi"("error in (no error)"=w448, "width"=sgl 26.0, "device"=w447) -> ("error out"=w464:errorcluster)  [unwired: 7 in, 1 out]
                n144 = local write "Cosmic Filter"(w402) -> ()
                n145 = call <userlib>:"AT Spectrograph Set Number Pixels.vi"("error in (no error)"=w464, "numberPixels"=1024, "device"=w447) -> ("error out"=w443:errorcluster)  [unwired: 7 in, 1 out]
                n146 = call <userlib>:"AT Spectrograph Get Grating.vi"("error in (no error)"=w443, "device"=w445) -> ("error out"=w442:errorcluster, "grating out"=w460:i32)  [unwired: 7 in, 1 out]
                "grating out" <- w460
                n147 = call <userlib>:"AT Spectrograph Get Grating Offset.vi"("error in (no error)"=w442, "grating"=w460, "device"=w445) -> ("error out"=w462:errorcluster, "offset out"=→"Grating offset":i32)  [unwired: 6 in, 1 out]
                n148 = call <userlib>:"AT Spectrograph Get Detector Offset.vi"("error in (no error)"=w462, "exitPort"=w459, "entrancePort"=w458, "device"=w445) -> ("error out"=w444:errorcluster, "offset out"=→"Detector offset":i32)  [unwired: 5 in, 1 out]
                n149 = call <userlib>:"AT Spectrograph Get Calibration.vi"("error in (no error)"=w444, "numberPixels"=1024, "device"=w445) -> ("error out"=w439:errorcluster, "calibrationValuesOut"=w436:sgl[])  [unwired: 5 in, 1 out]
                "CalValues" <- w436
                n150 = Bundle("wavelength out"=w437, "calibrationValuesOut"=w436, "gain"=w434, w433) -> (w435:T13)  [unwired: 1 in]
                n151 = Bundle By Name(cluster=T4 {"Message"="InitOp", "Data"=variant, "Code"=1}, "Data"=w435) -> (w441:T4)
                n152 = Enqueue Element(queue=w431, element=w441, error in (no error)=w439) -> (error out=w438:errorcluster)  [unwired: 1 in, 2 out]
                n153 = call-dynamic "SetClassQueueMessage.vi"("ErrorIn(No Error)"=w408, "Menu déroulant"=w429, "DefaultDev.lvclass"=w403) -> ("sortie d'erreur"=w407:errorcluster, "DefaultDev.lvclass Out"=w428:refnum<class "AndorSpectro.lvclass">)  [unwired: 7 in]
                n154 = Merge Errors(w407, w438) -> (w409:errorcluster)
                "Init Program" <- FALSE
              }
            }
          }
          event "Cosmic Filter": Value Change {
            n155 = event-data() -> ("NewVal"=w495:bool)  [unwired: 1 in, 5 out]
            n156 = case shown="Vrai" FALSE {
              frame False {
              }
              frame True {
                (unwired) u32 0 ("Mode")
                # "Vi for data avg filter and spurious filter"
                n157 = call <userlib>:"Filter_SetMode.vi"() -> ()  [unwired: 2 in, 2 out]
                n158 = call <userlib>:"Filter_GetMode.vi"() -> ()  [unwired: 1 in, 3 out]
                n159 = call <userlib>:"Filter_GetDataAveragingMode.vi"() -> ()  [unwired: 1 in, 3 out]
                n160 = call <userlib>:"Filter_GetThreshold.vi"() -> ()  [unwired: 1 in, 3 out]
                n161 = call <userlib>:"Filter_GetAveragingFactor.vi"() -> ()  [unwired: 1 in, 3 out]
                n162 = call <userlib>:"Filter_GetAveragingFrameCount.vi"() -> ()  [unwired: 1 in, 3 out]
                n163 = call <userlib>:"Filter_SetThreshold.vi"() -> ()  [unwired: 2 in, 2 out]
              }
            }
            n164 = Bundle By Name(cluster=cluster{"Message":string, "Data":variant, i32} {"Message"="SetCosmic", "Data"=variant, 0} ("ClassQueue"), "Data"=w495) -> (w496:cluster{"Message":string, "Data":variant, i32})
            n165 = call <userlib>:"SetFilterMode.vi"("error in (no error)"=w498, "mode"=w495) -> ("error out"=w494:errorcluster)  [unwired: 1 out]
            n166 = Enqueue Element(queue=w492, element=w496, error in (no error)=w494) -> (error out=w493:errorcluster)  [unwired: 1 in, 2 out]
          }
          event "HS": Value Change {
            n167 = event-data() -> ("NewVal"=w501:u16)  [unwired: 1 in, 5 out]
            n168 = call <userlib>:"SetHSSpeed.vi"("error in (no error)"=w505, "index"=w501, "type"=HSSpeed_type_typedef."EM Amp") -> ("error out"=w504:errorcluster)  [unwired: 1 in, 1 out]
            n169 = case shown="Vrai" TRUE {
              tunnel: w504 -> [w508 w512]
              tunnel: [w508 w519] -> w503
              tunnel: [_ w518] -> _
              tunnel: w501 -> [_ w515]
              tunnel: [_ w514] -> _
              tunnel: [_ w513] -> _
              tunnel: [_ w511] -> _
              tunnel: [_ w510] -> _
              tunnel: [_ w509] -> _
              frame False {
              }
              frame True {
                n170 = call <userlib>:"GetNumberHorizontalSpeeds.vi"("error in (no error)"=w512) -> ("number"=w513:dbl, "Dll Error Code"=w511:u32)  [unwired: 1 out]
                n171 = call <userlib>:"GetHSSpeed.vi"("error in (no error)"=w512, "index"=w515, "type"=HSSpeed_type_typedef."EM Amp", "channel"=0) -> ("error out"=w519:errorcluster, "DLL error code"=w509:u32, "speed"=w518:sgl)  [unwired: 1 in]
                n172 = call <userlib>:"GetHorizontalSpeed.vi"("index"=w515, "error in (no error)"=w512) -> ("speed"=w514:dbl, "Dll Error Code"=w510:u32)  [unwired: 1 out]
              }
            }
          }
          event "VS": Value Change {
            n173 = event-data() -> ("NewVal"=w522:u16)  [unwired: 1 in, 5 out]
            n174 = call <userlib>:"SetVSSpeed.vi"("error in (no error)"=w523, "index"=w522) -> ("error out"=w521:errorcluster)  [unwired: 1 out]
          }
          event "Accumulation": Value Change {
            n175 = event-data() -> ("NewVal"=w526:u16)  [unwired: 1 in]
            n176 = To Long Integer(number=w526) -> (32bit integer=w525:i32)
            n177 = Bundle By Name(cluster=T4 {"Message"="SetAccum", "Data"=variant, "Code"=0}, "Data"=w525) -> (w530:T4)
            n178 = Enqueue Element(queue=w524, element=w530, error in (no error)=w527) -> (error out=w528:errorcluster)  [unwired: 1 in, 2 out]
            n179 = local read "IntegTime"() -> (w531:u32)
            n180 = Bundle By Name(cluster=T4 {"Message"="SetInteg", "Data"=variant, "Code"=0}, "Data"=w531) -> (w533:T4)
            n181 = Enqueue Element(queue=w524, element=w533, error in (no error)=w528) -> (error out=w532:errorcluster)  [unwired: 1 in, 2 out]
          }
          event "Image Mode": Value Change {
            w549 = T12 1 items=["UpdateClassData", "UpdateMainClass", "UpdateDataBind", "ReInitDevice", "Custom", "ClosePan"] ("Menu déroulant")
            n182 = event-data() -> ("NewVal"=w539:bool)  [unwired: 1 in]
            n183 = local read "Y Bins"() -> (w547:i32)
            n184 = local read "Backgnd Mode"() -> (w544:T2)
            n185 = local read "WaveBands"() -> (w537:T3)
            n186 = Select(t=256 ("numAreas"), s=w539, f=w547) -> (s? t:f=w546:i32)
            n187 = Bundle By Name(cluster=T4 {"Message"="SetImMode", "Data"=variant, "Code"=0}, "Data"=w539) -> (w570:T4)
            n188 = Select(t=AndorNoiseCorr."Off" ("Backgnd Mode"), s=w539, f=w544) -> (s? t:f=w543:T2)
            n189 = local read "Accumulation"() -> (w562:u16)
            n190 = Enqueue Element(queue=w565, element=w570, error in (no error)=w558) -> (error out=w568:errorcluster)  [unwired: 1 in, 2 out]
            n191 = Select(t=T3 [] ("WaveBands"), s=w539, f=w537) -> (s? t:f=w536:T3)
            n192 = call <userlib>:"Andor Format CrvNames.vi"("WaveBands"=w536, "Background Mode"=w543, "NoiseWindow"=FALSE, "error in (no err)"=w558, "Accumulation"=1, "numAreas"=w546) -> ("error out"=w542:errorcluster, "DatDisplayNm"=w540:string[], "VarParY"=w551:dbl[], "SubDatDisplayNm"=w552:string[])  [unwired: 2 in]
            n193 = local write "Backgnd Mode"(w543) -> ()
            n194 = Bundle By Name(cluster=T4 {"Message"="SetAccum", "Data"=variant, "Code"=0}, "Data"=w562) -> (w563:T4)
            n195 = local read "IntegTime"() -> (w561:u32)
            n196 = Enqueue Element(queue=w565, element=w563, error in (no error)=w568) -> (error out=w567:errorcluster)  [unwired: 1 in, 2 out]
            n197 = property class="AndorSpectro.lvclass"(reference=w571, error in=w542, "Accessor:SubDatDisplayNm"=w552, "Accessor:SubScanTable(y)"=w551, "Accessor:ArrayDatNm"=w540) -> (reference out=w550:refnum<class "AndorSpectro.lvclass">, error out=w541:errorcluster)
            n198 = Bundle By Name(cluster=T4 {"Message"="SetInteg", "Data"=variant, "Code"=0}, "Data"=w561) -> (w559:T4)
            n199 = Enqueue Element(queue=w565, element=w559, error in (no error)=w567) -> (error out=w566:errorcluster)  [unwired: 1 in, 2 out]
            n200 = call-dynamic "SetClassQueueMessage.vi"("ErrorIn(No Error)"=w541, "Menu déroulant"=w549, "DefaultDev.lvclass"=w550) -> ("sortie d'erreur"=w555:errorcluster, "DefaultDev.lvclass Out"=w556:refnum<class "AndorSpectro.lvclass">)  [unwired: 7 in]
            n201 = Merge Errors(w555, w566) -> (w557:errorcluster)
          }
          event "Cont. Acq.": Value Change {
            n202 = event-data() -> ("NewVal"=w576:bool)  [unwired: 1 in, 5 out]
            n203 = case shown="Vrai" w576 {
              tunnel: w574 -> [w577 w591]
              tunnel: [w581 w590] -> w573
              tunnel: w572 -> [_ w589]
              frame False {
                n204 = local read "Accumulation"() -> (w580:u16)
                n205 = property on="Stop Acq" class="Bool (strict)"(error in=w577, "Value"=TRUE ("Stop Acq")) -> (error out=w578:errorcluster)  [unwired: 1 in, 1 out]
                n206 = property on="Accumulation" class="NumNb (strict)"(error in=w578, "Val(Sgnl)"=w580) -> (error out=w581:errorcluster)  [unwired: 1 in, 1 out]
              }
              frame True {
                n207 = call <userlib>:"SetAcquisitionMode.vi"("error in (no error)"=w591, "mode"=AcquisitionMode_mode_typedef."Run Till Abort") -> ("error out"=w587:errorcluster)  [unwired: 1 out]
                n208 = flat-sequence {
                  tunnel: [w593] -> w588
                  tunnel: w587 -> [w593]
                  frame #0 {
                    n209 = local write "Save Data"(FALSE ("Save Data")) -> ()
                  }
                }
                n210 = Bundle(FALSE, 0) -> (w586:cluster{bool, i32})  [unwired: 1 in]
                n211 = Bundle By Name(cluster=T4 {"Message"="Acquire", "Data"=variant, "Code"=0}, "Data"=w586) -> (w582:T4)
                n212 = Enqueue Element(queue=w589, element=w582, error in (no error)=w588) -> (error out=w590:errorcluster)  [unwired: 1 in, 2 out]
              }
            }
          }
          event "Background": Value Change {
            n213 = event-data() -> ("NewVal"=w596:i32[][])  [unwired: 1 in]
            n214 = Bundle By Name(cluster=T4 {"Message"="SetBckGnd", "Data"=variant, "Code"=0}, "Data"=w596) -> (w600:T4)
            n215 = Enqueue Element(queue=w597, element=w600, error in (no error)=w598) -> (error out=w595:errorcluster)  [unwired: 1 in, 2 out]
          }
          event "Acq": Value Change {
            n216 = event-data() -> ("NewVal"=w604:bool)  [unwired: 1 in, 5 out]
            n217 = case shown="Faux" w604 {
              tunnel: [w606 w622] -> w603
              tunnel: w602 -> [w608 w622]
              frame False {
                n218 = local read "Save Bckgnd"() -> (w607:bool)
                n219 = case shown="Vrai" w607 {
                  tunnel: w608 -> [w610 w619]
                  tunnel: [w610 w611] -> w606
                  frame False {
                    n220 = local write "Aquiring"(FALSE) -> ()
                  }
                  frame True {
                    w615 = 100 ("closingtime")
                    n221 = property on="Save Bckgnd" class="Bool (strict)"(error in=w619, "Val(Sgnl)"=FALSE ("Valeur (Signalisation)")) -> (error out=w617:errorcluster)  [unwired: 1 in, 1 out]
                    n222 = flat-sequence {
                      tunnel: [w621] -> w612
                      tunnel: w617 -> [w621]
                      frame #0 {
                        w620 = FALSE
                        n223 = local write "Cont. Acq."(w620) -> ()
                        n224 = local write "Aquiring"(w620) -> ()
                      }
                    }
                    n225 = local write "Shutter"(TRUE ("Shutter")) -> ()
                    n226 = call <userlib>:"SetShutter.vi"("type"=Shutter_type_typedef."TTL High", "mode"=Shutter_mode_typedef."Open", "closingtime"=w615, "openingtime"=w615, "error in (no error)"=w612) -> ("error out"=w611:errorcluster)  [unwired: 9 in, 1 out]
                  }
                }
              }
              frame True {
              }
            }
          }
          event Value Change {
            w630 = T12 1 items=["UpdateClassData", "UpdateMainClass", "UpdateDataBind", "ReInitDevice", "Custom", "ClosePan"] ("Menu déroulant")
            n227 = event-data() -> ("NewVal"=w640:T2)  [unwired: 1 in, 1 out]
            n228 = local read "Background"() -> (w637:i32[][])
            n229 = local read "WaveBands"() -> (w624:T3)
            n230 = Empty Array?(array=w637) -> (empty?=w625:bool)
            n231 = case shown="Vrai" w625 {
              frame False {
              }
              frame True {
                n232 = One Button Dialog(message="No valid background data available. Please acquire Background") -> ()  [unwired: 1 in, 1 out]
              }
            }
            n233 = call <userlib>:"Andor Format CrvNames.vi"("WaveBands"=w624, "Background Mode"=w640, "NoiseWindow"=FALSE, "error in (no err)"=w641, "Accumulation"=1, "numAreas"=1) -> ("error out"=w627:errorcluster, "DatDisplayNm"=w623:string[], "VarParY"=w628:dbl[], "SubDatDisplayNm"=w629:string[])  [unwired: 2 in]
            n234 = Bundle By Name(cluster=T4 {"Message"="SetBckGndMode", "Data"=variant, "Code"=0}, "Data"=w640) -> (w635:T4)
            n235 = property class="AndorSpectro.lvclass"(reference=w639, error in=w627, "Accessor:SubDatDisplayNm"=w629, "Accessor:SubScanTable(y)"=w628, "Accessor:ArrayDatNm"=w623) -> (reference out=w631:refnum<class "AndorSpectro.lvclass">, error out=w626:errorcluster)
            n236 = Enqueue Element(queue=w643, element=w635, error in (no error)=w641) -> (error out=w642:errorcluster)  [unwired: 1 in, 2 out]
            n237 = call-dynamic "SetClassQueueMessage.vi"("ErrorIn(No Error)"=w626, "Menu déroulant"=w630, "DefaultDev.lvclass"=w631) -> ("DefaultDev.lvclass Out"=w638:refnum<class "AndorSpectro.lvclass">)  [unwired: 7 in, 1 out]
          }
          event "Shutter": Value Change {
            w648 = 100 ("closingtime")
            n238 = event-data() -> ("NewVal"=w652:bool)  [unwired: 1 in, 5 out]
            n239 = Not(x=w652) -> (.not. x?=w645:bool)
            n240 = Select(t=Shutter_mode_typedef."Close" ("mode"), s=w645, f=Shutter_mode_typedef."Open" ("mode")) -> (s? t:f=w649:T5)
            n241 = call <userlib>:"SetShutter.vi"("type"=Shutter_type_typedef."TTL High", "mode"=w649, "closingtime"=w648, "openingtime"=w648, "error in (no error)"=w647) -> ("error out"=w646:errorcluster)  [unwired: 9 in, 1 out]
          }
          event "Save Bckgnd": Value Change {
            w673 = T12 1 items=["UpdateClassData", "UpdateMainClass", "UpdateDataBind", "ReInitDevice", "Custom", "ClosePan"] ("Menu déroulant")
            n242 = event-data() -> ("NewVal"=w663:bool)  [unwired: 1 in, 5 out]
            n243 = local read "Backgnd Mode"() -> (w662:T2)
            n244 = local read "WaveBands"() -> (w661:T3)
            n245 = Select(t=AndorNoiseCorr."Off" ("Backgnd Mode"), s=w663, f=w662) -> (s? t:f=w658:T2)
            n246 = call <userlib>:"Andor Format CrvNames.vi"("WaveBands"=w661, "Background Mode"=w658, "NoiseWindow"=FALSE, "error in (no err)"=w665, "Accumulation"=1, "numAreas"=1) -> ("error out"=w670:errorcluster, "DatDisplayNm"=w668:string[], "VarParY"=w671:dbl[], "SubDatDisplayNm"=w672:string[])  [unwired: 2 in]
            n247 = Bundle By Name(cluster=T4 {"Message"="SetBckGndMode", "Data"=variant, "Code"=0}, "Data"=w658) -> (w659:T4)
            n248 = property class="AndorSpectro.lvclass"(reference=w667, error in=w670, "Accessor:SubDatDisplayNm"=w672, "Accessor:SubScanTable(y)"=w671, "Accessor:ArrayDatNm"=w668) -> (reference out=w674:refnum<class "AndorSpectro.lvclass">, error out=w669:errorcluster)
            n249 = call-dynamic "SetClassQueueMessage.vi"("ErrorIn(No Error)"=w669, "Menu déroulant"=w673, "DefaultDev.lvclass"=w674) -> ("sortie d'erreur"=w657:errorcluster, "DefaultDev.lvclass Out"=w666:refnum<class "AndorSpectro.lvclass">)  [unwired: 7 in]
            n250 = Enqueue Element(queue=w656, element=w659, error in (no error)=w657) -> (error out=w655:errorcluster)  [unwired: 1 in, 2 out]
          }
          event "WaveBands": Value Change {
            w686 = T12 1 items=["UpdateClassData", "UpdateMainClass", "UpdateDataBind", "ReInitDevice", "Custom", "ClosePan"] ("Menu déroulant")
            n251 = event-data() -> ("NewVal"=w680:T3)  [unwired: 1 in, 5 out]
            n252 = local read "Backgnd Mode"() -> (w679:T2)
            n253 = call <userlib>:"Andor Format CrvNames.vi"("WaveBands"=w680, "Background Mode"=w679, "NoiseWindow"=FALSE, "error in (no err)"=w693, "Accumulation"=1, "numAreas"=1) -> ("error out"=w683:errorcluster, "DatDisplayNm"=w681:string[], "VarParY"=w684:dbl[], "SubDatDisplayNm"=w685:string[])  [unwired: 2 in]
            n254 = property class="AndorSpectro.lvclass"(reference=w692, error in=w683, "Accessor:SubDatDisplayNm"=w685, "Accessor:SubScanTable(y)"=w684, "Accessor:ArrayDatNm"=w681) -> (reference out=w687:refnum<class "AndorSpectro.lvclass">, error out=w682:errorcluster)
            n255 = call-dynamic "SetClassQueueMessage.vi"("ErrorIn(No Error)"=w682, "Menu déroulant"=w686, "DefaultDev.lvclass"=w687) -> ("sortie d'erreur"=w678:errorcluster, "DefaultDev.lvclass Out"=w691:refnum<class "AndorSpectro.lvclass">)  [unwired: 7 in]
          }
          event "Cooler": Value Change {
            n256 = event-data() -> ("NewVal"=w696:bool)  [unwired: 1 in, 5 out]
            n257 = case shown="Vrai" w696 {
              tunnel: w695 -> [w699 w701]
              tunnel: [w698 w700] -> w694
              frame False {
                n258 = call <userlib>:"CoolerOFF.vi"("error in (no error)"=w699) -> ("error out"=w698:errorcluster)  [unwired: 1 in, 1 out]
              }
              frame True {
                n259 = call <userlib>:"CoolerON.vi"("error in (no error)"=w701) -> ("error out"=w700:errorcluster)  [unwired: 1 in, 1 out]
              }
            }
          }
          event "IntegTime": Value Change {
            n260 = event-data() -> ("NewVal"=w706:u32)  [unwired: 1 in, 5 out]
            n261 = Bundle By Name(cluster=T4 {"Message"="SetInteg", "Data"=variant, "Code"=0}, "Data"=w706) -> (w703:T4)
            n262 = Enqueue Element(queue=w709, element=w703, error in (no error)=w708) -> (error out=w705:errorcluster)  [unwired: 1 in, 2 out]
            n263 = Enqueue Element(queue=w704, element=w703, error in (no error)=w705) -> (error out=w702:errorcluster)  [unwired: 1 in, 2 out]
          }
          event "AquireImage": Value Change {
            n264 = event-data() -> ("NewVal"=w719:bool)  [unwired: 1 in]
            n265 = case shown="Vrai" w719 {
              tunnel: w718 -> [w720 w736]
              tunnel: w717 -> [w721 w727]
              tunnel: w716 -> [_ w734]
              tunnel: w715 -> [_ w735]
              tunnel: [w720 w733] -> w714
              tunnel: [w721 w731] -> w713
              tunnel: w712 -> [_ w726]
              tunnel: w711 -> [_ _]
              frame False {
              }
              frame True {
                n266 = local read "Save Bckgnd"() -> (w722:bool)
                n267 = local read "Save Data"() -> (w723:bool)
                n268 = property class="AndorSpectro.lvclass"(reference=w736, error in=w727) -> (reference out=w733:refnum<class "AndorSpectro.lvclass">, error out=w732:errorcluster, "Accessor:Function"=w741:string, "Accessor:InstrumentName"=w739:string)
                n269 = local read "Image Mode"() -> (w725:bool)
                n270 = Concatenate Strings(w741, "@" ("chaîne"), w739) -> (w737:string)
                n271 = Or(x=w722, y=w723) -> (x .or. y?=w724:bool)
                n272 = Bundle(w737, w724) -> (w738:cluster{string, bool})  [unwired: 1 in]
                n273 = case shown="Vrai" w724 {
                  tunnel: w738 -> [_ w757]
                  tunnel: w735 -> [_ w756]
                  tunnel: w734 -> [_ w755]
                  tunnel: w732 -> [w751 w754]
                  tunnel: [w750 w753] -> w731
                  tunnel: w726 -> [w752 _]
                  tunnel: w725 -> [w748 _]
                  frame False {
                    n274 = Bundle(FALSE, 0) -> (w745:cluster{bool, i32})  [unwired: 1 in]
                    n275 = Bundle By Name(cluster=T4 {"Message"="Acquire", "Data"=variant, "Code"=0}, "Data"=w745) -> (w743:T4)
                    n276 = Select(t=T4 {"Message"="AcquireIm", "Data"=variant, "Code"=0}, s=w748, f=w743) -> (s? t:f=w747:T4)
                    n277 = Enqueue Element(queue=w752, element=w747, error in (no error)=w751) -> (error out=w750:errorcluster)  [unwired: 1 in, 2 out]
                  }
                  frame True {
                    n278 = To Variant(anything=w757) -> (Variant=w760:variant)
                    n279 = Bundle By Name(cluster=cluster{"Message":string, "Data":variant, i32} {"Message"="ArrayDevAcqSetup", "Data"=variant, 0} ("élément"), "Data"=w760) -> (w759:cluster{"Message":string, "Data":variant, i32})
                    n280 = Enqueue Element(queue=w755, element=w759, error in (no error)=w754) -> (queue out=w762:refnum<queue>, error out=w758:errorcluster)  [unwired: 1 in, 1 out]
                    n281 = Generate User Event(user event=w756, event data cluster=w762, error in=w758) -> (error out=w753:errorcluster)  [unwired: 1 in, 1 out]
                  }
                }
                n282 = call <userlib>:"Wait_At_Wire_Bool.vi"("Wait (ms)"=u32 300, "error in (no error)"=FALSE) -> ("error out"=w729:bool)  [unwired: 7 in, 2 out]
                n283 = local write "AquireImage"(w729) -> ()
              }
            }
          }
          event "SetAreas": Value Change {
            w763 = 1 ("y")
            n284 = event-data() -> ()  [unwired: 1 in, 6 out]
            n285 = local read "Y End"() -> (w768:i32)
            n286 = local read "Y Start"() -> (w769:i32)
            n287 = local read "Y Bins"() -> (w770:i32)
            n288 = Greater?(x=w770, y=w763) -> (0:w767:bool)
            n289 = case shown="Faux" w767 {
              tunnel: w769 -> [w771 _]
              tunnel: w768 -> [w788 _]
              tunnel: w765 -> [w775 w789]
              tunnel: [w773 w789] -> w764
              tunnel: w763 -> [w780 _]
              frame False {
                n290 = Subtract(x=w788, y=w771) -> (x-y=w787:i32)
                n291 = Increment(x=w787) -> (x+1=w783:i32)
                n292 = call <userlib>:"SetReadMode.vi"("error in (no error)"=w775, "mode"=ReadMode_mode_typedef."Single-Track") -> ("error out"=w774:errorcluster)  [unwired: 1 out]
                n293 = Quotient & Remainder(x=w783, y=2) -> (floor(x/y)=w785:i32)  [unwired: 1 out]
                n294 = Add(x=w771, y=w785) -> (x+y=w784:i32)
                n295 = call <userlib>:"SetSingleTrack.vi"("error in (no error)"=w774, "height"=w783, "centre"=w784) -> ("error out"=w773:errorcluster)  [unwired: 1 in, 1 out]
                n296 = Build Array(w780, 0 ("élément"), w771, 1024 ("élément"), w783, w780, w780) -> (w777:i32[])
                n297 = Insert Into Array(array=i32[][] [] ("areas"), index (col)=0 ("indice désactivé (col)"), new element=w777) -> (w776:i32[][])  [unwired: 1 in]
                n298 = local write "areas"(w776) -> ()
              }
              frame True {
              }
            }
          }
          event "Gain": Value Change {
            n299 = event-data() -> ("NewVal"=w796:i32)  [unwired: 1 in]
            n300 = Bundle By Name(cluster=cluster{"Message":string, "Data":variant, i32} {"Message"="SetGain", "Data"=variant, 0} ("ClassQueue"), "Data"=w796) -> (w792:cluster{"Message":string, "Data":variant, i32})
            n301 = Enqueue Element(queue=w794, element=w792, error in (no error)=w795) -> (error out=w791:errorcluster)  [unwired: 1 in, 2 out]
            n302 = Enqueue Element(queue=w793, element=w792, error in (no error)=w791) -> (error out=w790:errorcluster)  [unwired: 1 in, 2 out]
          }
        }
      }
      n303 = while {
        shift-right: [w45] -> w19
        shift-left: w22 -> [w46]
        shift-right: [w42] -> _
        shift-left: w24 -> [w40]
        tunnel: w17 -> [w37]
        tunnel: [w37] -> w9
        tunnel: w14 -> [w36]
        stop <- w39 stop-if-true
        n304 = Dequeue Element(queue=w46, error in (no error)=w40) -> (queue out=w45:refnum<queue>, element=w44:T4, error out=w41:errorcluster)  [unwired: 1 in, 1 out]
        n305 = Unbundle By Name(w44) -> ("Message"=w43:string, "Data"=w38:variant, "Code"=w35:i32)
        n306 = case shown="\"Acquire\"" w43 {
          tunnel: [w47 w51 w61 w130 w141 w149 w153 w170 w180 w191] -> w42
          tunnel: w41 -> [w49 w51 w66 w128 w143 w151 w156 w177 w180 w195]
          tunnel: [_ TRUE _ _ _ _ _ _ _ _] -> w39
          tunnel: w38 -> [_ _ w59 _ w146 w152 w158 w179 _ w200]
          tunnel: w37 -> [_ _ w82 w136 _ _ _ _ _ _]
          tunnel: w36 -> [_ _ w81 w135 _ _ _ _ _ _]
          tunnel: w35 -> [_ _ w80 w134 _ _ _ _ _ _]
          tunnel: [_ _ _ _ _ _ _ _ _ w198] -> _
          tunnel: [_ _ _ _ _ _ _ _ _ w197] -> _
          tunnel: [_ _ _ _ _ _ _ _ _ w196] -> _
          tunnel: [_ _ _ _ _ _ _ _ _ w187] -> _
          tunnel: [_ _ _ _ _ _ _ _ _ w183] -> _
          frame "Error", Default {
            n307 = call <vilib>:"General Error Handler.vi"("error in (no error)"=w49) -> ("error out"=w48:errorcluster)  [unwired: 10 in, 4 out]
            n308 = call <vilib>:"Clear Errors.vi"("error in (no error)"=w48) -> ("error out"=w47:errorcluster)  [unwired: 5 in, 1 out]
          }
          frame "Stop" {
          }
          frame "Acquire" {
            n309 = Not Equal To 0?(x=w80) -> (x != 0?=w55:bool)
            n310 = local read "Accumulation"() -> (w72:u16)
            n311 = local read "Cont. Acq."() -> (w71:bool)
            n312 = local read "Save Bckgnd"() -> (w68:bool)
            n313 = flat-sequence {
              tunnel: [w117] -> w77
              tunnel: w66 -> [w117]
              frame #0 {
                n314 = local write "Aquiring"(TRUE) -> ()
              }
            }
            n315 = local read "Shutter"() -> (w53:bool)
            n316 = And(x=w68, y=w53) -> (x .and. y?=w54:bool)
            n317 = case shown="Vrai" w54 {
              selector: w54 -> [w89 w98]
              tunnel: [w89 w98] -> w67
              tunnel: w66 -> [w88 w93]
              tunnel: [w88 w91] -> w64
              frame False {
              }
              frame True {
                w97 = 100 ("closingtime")
                n318 = call <userlib>:"SetShutter.vi"("type"=Shutter_type_typedef."TTL High", "mode"=Shutter_mode_typedef."Close", "closingtime"=w97, "openingtime"=w97, "error in (no error)"=w93) -> ("error out"=w94:errorcluster)  [unwired: 9 in, 1 out]
                n319 = local write "Shutter"(FALSE ("Shutter")) -> ()
                n320 = call <userlib>:"Wait_At_Wire_Err.vi"("Wait (ms)"=u32 200, "error in (no error)"=w94) -> ("error out"=w91:errorcluster)  [unwired: 7 in, 2 out]
              }
            }
            n321 = Select(t=u16 10000 ("cas vrai"), s=w71, f=w72) -> (s? t:f=w69:u16)
            n322 = Variant To Data(type=cluster{"Scan":bool, "CurvePointIndex":i32} {"Scan"=TRUE, "CurvePointIndex"=0} ("Settings"), Variant=w59) -> (data=w57:cluster{"Scan":bool, "CurvePointIndex":i32})  [unwired: 1 in, 1 out]
            n323 = local read "Cosmic Filter"() -> (w52:bool)
            n324 = local read "IntegTime"() -> (w78:u32)
            n325 = control-ref of="Stop Acq"() -> (w79:refnum<vi>)
            n326 = control-ref of="AccDone"() -> (w74:refnum<vi>)
            n327 = Or(x=w67, y=w55) -> (x .or. y?=w73:bool)
            n328 = Merge Errors(w64, w77) -> (w65:errorcluster)
            n329 = local read "Save Bckgnd"() -> (w76:bool)
            n330 = call <userlib>:"Andor_Acquire.vi"("AndorAcqQ"=w81, "Accumulation"=w69, "IntegTime"=w78, "AndorOpQ"=w82, "Save"=w73, "CosmicFilter"=w52, "ErrorIn(NoErr)"=w65, "Stop Acq"=w79, "AccDoneRef"=w74) -> ("Data out"=w75:i32[], "error out"=w63:errorcluster)  [unwired: 4 in, 1 out]
            n331 = Unbundle By Name(w57) -> ("Scan"=w56:bool)
            n332 = case shown="Vrai" w76 {
              tunnel: w75 -> [_ w107]
              tunnel: w63 -> [w99 w105]
              tunnel: [w99 w104] -> w60
              tunnel: w57 -> [_ w106]
              tunnel: w56 -> [_ w102]
              frame False {
              }
              frame True {
                n333 = call <userlib>:"Andor_ProcessBckgnd.vi"("error in (no error)"=w105, "Settings"=w106, "BackgroundIn"=w107) -> ("error out"=w101:errorcluster, "BackgroundOut"=w103:i32[][])  [unwired: 7 in]
                n334 = case shown="Faux" w102 {
                  tunnel: w101 -> [w111 w116]
                  tunnel: [w108 w116] -> w100
                  frame False {
                    w112 = 100 ("closingtime")
                    n335 = local write "Shutter"(TRUE ("Shutter")) -> ()
                    n336 = call <userlib>:"SetShutter.vi"("type"=Shutter_type_typedef."TTL High", "mode"=Shutter_mode_typedef."Open", "closingtime"=w112, "openingtime"=w112, "error in (no error)"=w111) -> ("error out"=w110:errorcluster)  [unwired: 9 in, 1 out]
                    n337 = property on="Save Bckgnd" class="Bool (strict)"(error in=w110, "Val(Sgnl)"=FALSE ("Save Bckgnd")) -> (error out=w108:errorcluster)  [unwired: 1 in, 1 out]
                  }
                  frame True {
                  }
                }
                n338 = property on="Background" class="Tabl (strict)"(error in=w100, "Val(Sgnl)"=w103) -> (error out=w104:errorcluster)  [unwired: 1 in, 1 out]
              }
            }
            n339 = case shown="Vrai" w56 {
              tunnel: w63 -> [w84 w87]
              tunnel: [w83 w87] -> w62
              frame False {
                n340 = flat-sequence {
                  tunnel: [w86] -> w83
                  tunnel: w84 -> [w86]
                  frame #0 {
                    w85 = FALSE
                    n341 = local write "Cont. Acq."(w85) -> ()
                    n342 = local write "Aquiring"(w85) -> ()
                  }
                }
              }
              frame True {
              }
            }
            n343 = Merge Errors(w60, w62) -> (w61:errorcluster)
          }
          frame "AcquireIm" {
            n344 = flat-sequence {
              tunnel: [w137] -> w127
              tunnel: w128 -> [w137]
              frame #0 {
                n345 = local write "Aquiring"(TRUE) -> ()
              }
            }
            n346 = Not Equal To 0?(x=w134) -> (x != 0?=w133:bool)
            n347 = local read "Save Bckgnd"() -> (w124:bool)
            n348 = local read "Accumulation"() -> (w123:u16)
            n349 = local read "Cont. Acq."() -> (w122:bool)
            n350 = Or(x=w124, y=w133) -> (x .or. y?=w125:bool)
            n351 = Select(t=u16 10000 ("cas vrai"), s=w122, f=w123) -> (s? t:f=w120:u16)
            n352 = local read "IntegTime"() -> (w131:u32)
            n353 = control-ref of="Stop Acq"() -> (w132:refnum<vi>)
            n354 = control-ref of="AccDone"() -> (w126:refnum<vi>)
            n355 = call <userlib>:"Andor_Acquire_Im.vi"("AccDoneRef"=w126, "IntegTime"=w131, "Stop Acq"=w132, "Accumulation"=w120, "ErrorIn(NoErr)"=w127, "Save"=w125, "AndorOpQ"=w136, "AndorAcqQ"=w135) -> ("error out"=w129:errorcluster, "Data out"=w119:i32[][])  [unwired: 2 out]
            n356 = flat-sequence {
              tunnel: [w140] -> w130
              tunnel: w129 -> [w140]
              tunnel: w119 -> [_]
              frame #0 {
                w139 = FALSE
                n357 = local write "Cont. Acq."(w139) -> ()
                n358 = local write "Aquiring"(w139) -> ()
              }
            }
          }
          frame "SetGain" {
            n359 = Variant To Data(error in=w143, type=0, Variant=w146) -> (data=w144:i32, error out=w142:errorcluster)
            n360 = call <userlib>:"SetPreAmpGain.vi"("error in (no error)"=w142, "index"=w144) -> ("error out"=w141:errorcluster)  [unwired: 1 out]
          }
          frame "SetCosmic" {
            n361 = Variant To Data(error in=w151, type=TRUE, Variant=w152) -> (data=w147:bool, error out=w148:errorcluster)
            n362 = call <userlib>:"SetFilterMode.vi"("error in (no error)"=w148, "mode"=w147) -> ("error out"=w149:errorcluster)  [unwired: 1 out]
          }
          frame "SetAccum" {
            n363 = Variant To Data(error in=w156, type=0, Variant=w158) -> (data=w155:i32, error out=w154:errorcluster)
            n364 = case shown="Par défaut" w155 {
              selector: w155 -> [w159 _]
              tunnel: w154 -> [w163 w166]
              tunnel: [w160 w165] -> w153
              frame Default {
                n365 = call <userlib>:"SetAcquisitionMode.vi"("error in (no error)"=w163, "mode"=AcquisitionMode_mode_typedef."Accumulate") -> ("error out"=w161:errorcluster)  [unwired: 1 out]
                n366 = call <userlib>:"SetNumberAccumulations.vi"("error in (no error)"=w161, "number"=w159) -> ("error out"=w160:errorcluster)  [unwired: 1 out]
              }
              frame 1 {
                # "Single scan mode"
                n367 = call <userlib>:"SetAcquisitionMode.vi"("error in (no error)"=w166, "mode"=AcquisitionMode_mode_typedef."Single Scan") -> ("error out"=w165:errorcluster)  [unwired: 1 out]
              }
            }
          }
          frame "SetImMode" {
            w168 = 1 ("hbin")
            n368 = Variant To Data(error in=w177, type=TRUE, Variant=w179) -> (data=w172:bool, error out=w176:errorcluster)
            n369 = Select(t=ReadMode_mode_typedef."Image" ("mode"), s=w172, f=ReadMode_mode_typedef."Full Vertical Binning" ("mode")) -> (s? t:f=w173:T8)
            n370 = call <userlib>:"SetReadMode.vi"("error in (no error)"=w176, "mode"=w173) -> ("error out"=w171:errorcluster)  [unwired: 1 out]
            n371 = call <userlib>:"SetImage.vi"("hbin"=w168, "vbin"=w168, "hstart"=w168, "hend"=1024, "vstart"=w168, "vend"=256, "error in (no error)"=w171) -> ("error out"=w170:errorcluster)  [unwired: 19 in, 1 out]
          }
          frame "AcquireLive" {
          }
          frame "SetInteg" {
            n372 = Variant To Data(type=u32 0, Variant=w200) -> (data=w199:u32)  [unwired: 1 in, 1 out]
            n373 = To Single Precision Float(number=w199) -> (single precision float=w202:sgl)
            n374 = Divide(x=w202, y=sgl 1000.0) -> (x/y=w189:sgl)
            n375 = call <userlib>:"SetExposureTime.vi"("error in (no error)"=w195, "time"=w189) -> ("error out"=w193:errorcluster, "DLL error code"=w197:u32)
            n376 = local read "Accumulation"() -> (w186:u16)
            n377 = call <userlib>:"SetAccumulationCycleTime.vi"("error in (no error)"=w193, "time"=w189) -> ("error out"=w194:errorcluster, "DLL error code"=w198:u32)
            n378 = Greater?(x=w186, y=u16 1) -> (0:w181:bool)
            n379 = call <userlib>:"GetAcquisitionTimings.vi"("exposure input"=w189, "accumulate input"=w186, "error in (no error)"=w194) -> ("exposure"=→"exposure":sgl, "accumulate"=w182:sgl, "DLL error code"=w196:u32, "error out"=w192:errorcluster)  [unwired: 8 in, 1 out]
            n380 = call <userlib>:"GetReadOutTime.vi"("error in (no error)"=w192) -> ("error out"=w191:errorcluster, "readOutTime"=w187:sgl)  [unwired: 4 in, 1 out]
            n381 = Add(x=w189, y=w187) -> (x+y=w188:sgl)
            n382 = Multiply(x=w188, y=w186) -> (x*y=w183:sgl)
            n383 = Select(t=w183, s=w181, f=w182) -> (s? t:f=w184:sgl)
            n384 = local write "AcqTime"(w184) -> ()
          }
        }
      }
      n385 = Release Queue(queue=w9, error in (no error)=w8) -> ()  [unwired: 1 in, 3 out]
      n386 = Release Queue(queue=w19, error in (no error)=w8) -> ()  [unwired: 1 in, 3 out]
    }
    frame Error {
    }
  }
  "error out" <- w5
  "AndorSpectro.lvclass Out" <- w3
